vi "InitAction.vi"(6 "InstrumentName":string, 7 "VisaRessIn":refnum<visa-resource-name>, 8 "error in (no error)":errorcluster caption="entrée d'erreur (pas d'erreur)", 9 "FirstClassInst":bool, 10 "Function":string, 11 "GenData In":refnum<class "Tools.lvclass"> caption="DNL_LabVIEW Object in") -> (0 "error out":errorcluster caption="sortie d'erreur", 3 "GenData Out":refnum<class "Tools.lvclass"> caption="DNL_LabVIEW Object out")   [LabVIEW 2019, in "Tools.lvclass"]
uses:
  Tools.lvclass
  Tools_Func.ctl
  Tools.lvclass/Tools.ctl
panel:
  in  "GenData_Func":T1=enum."Courbe 2 (Arb)"
  out "VisaRessOut":refnum<visa-resource-name>
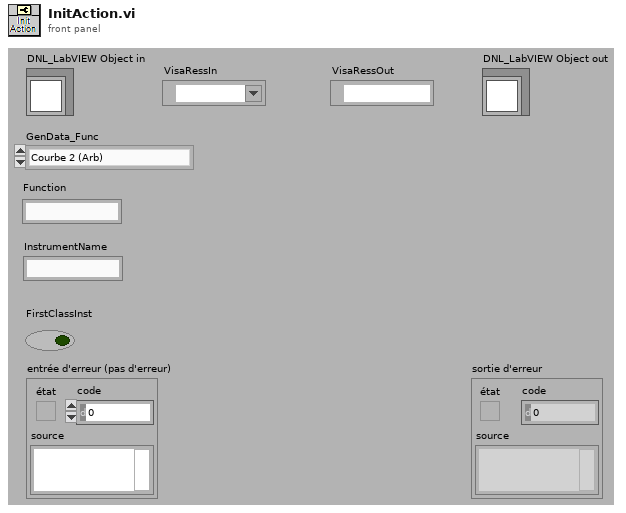
[diagram p1: front panel]
types:
  T1 = typedef "Tools.lvclass/Tools_Func.ctl" = enum16{"Courbe 1 (Arb)", "Courbe 2 (Arb)", "Courbe 3 (Arb)", "Courbe 123 (Arb,Arb,Arb)", "Scan Pos (Arb)", "Indice de Point (Points)", "AbsTime (ms)", "Minuteur (s)", "Panneaux Infos (Na)", "Délais (ms)", "RandwithDbind(Arb)", "RandomNum (Arb)", "Multisweep (Sw)", "ScanTime (s)"}
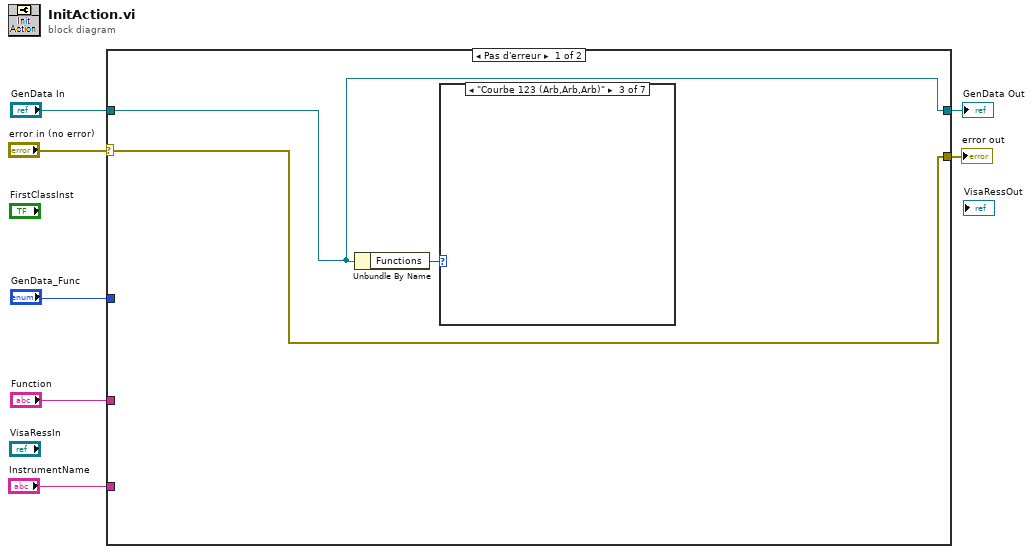
[diagram p0: block diagram]
diagram:
  n1 = case shown="Pas d'erreur" "error in (no error)" {
    selector: "error in (no error)" -> [w8 w12]
    tunnel: [w8 w12] -> w6
    tunnel: "GenData In" -> [w9 w11]
    tunnel: [w9 w11] -> w4
    tunnel: "GenData_Func" -> [_ _]
    tunnel: "Function" -> [_ _]
    tunnel: "InstrumentName" -> [_ _]
    frame No Error {
      n2 = Unbundle By Name(w9) -> ("Functions"=w10:T1)
      n3 = case shown="\"Courbe 123 (Arb,Arb,Arb)\"" w10 {
        frame "Courbe 1 (Arb)" {
        }
        frame "Courbe 2 (Arb)" {
        }
        frame "Courbe 123 (Arb,Arb,Arb)" {
        }
        frame "Indice de Point (Points)" {
        }
        frame "Minuteur (s)" {
        }
        frame "Délais (ms)", Default {
        }
        frame "AbsTime (ms)" {
        }
      }
    }
    frame Error {
    }
  }
  "error out" <- w6
  "GenData Out" <- w4
